vi "COMI Write Mem Port DW.vi"(7 "dwOutVal":u32, 9 "nOffset":u32, 10 "dwPortBase":u32, 11 "hDevice":u32) -> (3 "hDevice out":u32)   [LabVIEW 2017, in "Comidll.lvlib"]
doc: "void (COMI_WriteMemPortDW) (HANDLE hDevice, unsigned long dwPortBase, unsigned long nOffset, unsigned long dwOutVal);"
uses:
  <userlib>/Comidll/Comidll.lvlib
  <userlib>/Comidll/Comidll.dll
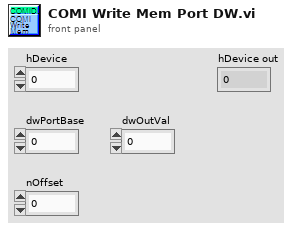
[diagram p1: front panel]
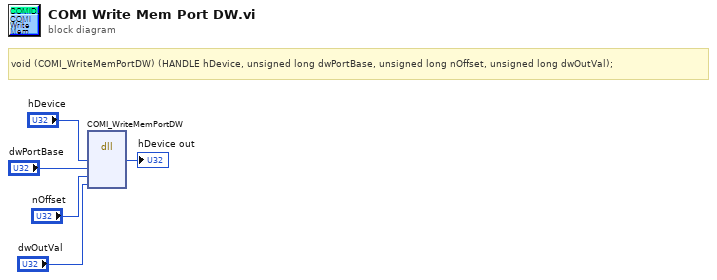
[diagram p0: block diagram]
diagram:
  # "void\t(COMI_WriteMemPortDW) (HANDLE hDevice, unsigned long dwPortBase, unsigned long nOffset, unsigned long dwOutVal);"
  n1 = dll-call lib="C:/Program Files/National Instruments/LabVIEW 2017/user.lib/Comidll/Comidll.*" fn="COMI_WriteMemPortDW"("hDevice"="hDevice", "dwPortBase"="dwPortBase", "nOffset"="nOffset", "dwOutVal"="dwOutVal") -> ("hDevice"=→"hDevice out":u32)  [unwired: 7 in, 2 out]
